vi "Write Cycle.vi"(0 "SRL Data Out":u8[][](array[numeric]) format="%.0x", 5 "Socket Mask":u32=1 format="%06x", 11 "error in":errorcluster, 13 "Log (T)":bool=TRUE, 14 "FPGA":T1) -> (15 "error out":errorcluster)   [LabVIEW 2017, in "Host SRL.lvlib"]
uses:
  Host SRL.lvlib
  Type Defs/WSVCAP SHL FPGA Enum.ctl
  Type Defs/WSVCAP SHL Function Enum.ctl
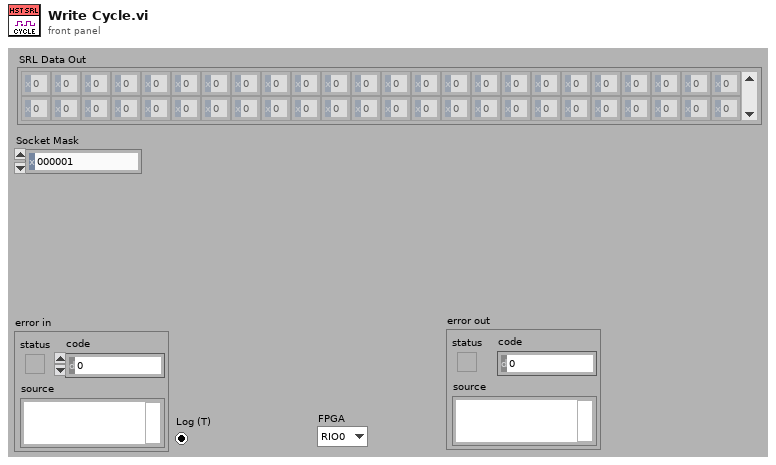
[diagram p1: front panel]
types:
  T1 = typedef "WSVCAP SHL FPGA Enum.ctl" = enum16{"RIO0", "RIO1"}
  T2 = typedef "WSVCAP SHL Function Enum.ctl" = enum16{"Initialize", "Configure I2C", "Configure SRL", "Write I2C", "Read I2C", "Write SRL", "Start SRL Cycle", "Stop SRL Cycle", "Get Status", "Close"}
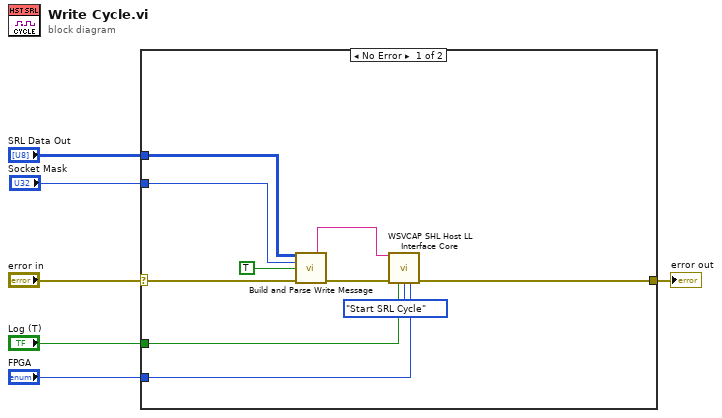
[diagram p0: block diagram]
diagram:
  n1 = case shown="No Error" "error in" {
    selector: "error in" -> [w13 w17]
    tunnel: [w9 w17] -> w6
    tunnel: "SRL Data Out" -> [w12 _]
    tunnel: "Socket Mask" -> [w10 _]
    tunnel: "Log (T)" -> [w11 _]
    tunnel: "FPGA" -> [w8 _]
    frame No Error {
      n2 = call "Build and Parse Write Message.vi"("Write Data In [DUT Ordered]"=w12, "Socket Mask [U32] In"=w10, "Cycle Mode In"=TRUE, "error in"=w13) -> ("Message Out"=w14:string, "error out"=w15:errorcluster)  [unwired: 6 in, 4 out]
      n3 = call "WSVCAP SHL Host LL Interface Core.vi"("Message In"=w14, "error in"=w15, "Log (T)"=w11, "Function"=WSVCAP_SHL_Function_Enum."Start SRL Cycle", "FPGA"=w8) -> ("error out"=w9:errorcluster)  [unwired: 8 in, 2 out]
    }
    frame Error {
    }
  }
  "error out" <- w6
